vi "open_project_Dialog.vi"(8 "error in (no error)":cluster{"状态":bool, "代码":i32, "源":string} caption="错误输入（无错误）", 11 "当前项目配置 输入":T1) -> (0 "error out":cluster{"状态":bool, "代码":i32, "源":string} caption="错误输出", 1 "结果":bool, 2 "取消？":bool, 3 "当前项目配置 输出":T1)   [LabVIEW 2018, in "menu.lvlib"]
uses:
  menu.lvlib
panel:
  in  "取消按钮":bool
  in  "确定按钮":bool
  in  "项目文件路径":path
  in  "项目名":string
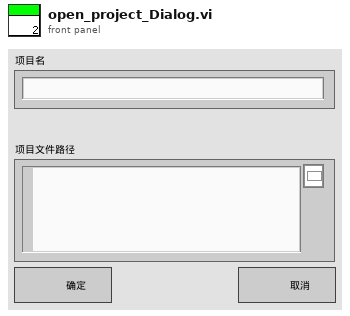
[diagram p1: front panel]
types:
  T1 = cluster{"控制参数配置":string, "模拟响应配置":string, "串口通信配置":string, "数据显示配置":string, "数据记录配置":string, "安全/报警配置":string, "模拟负载数据":string, "模拟加载数据":string, "总电源":bool, "电机1上电":bool, "电机2上电":bool, "串口连接":bool, "电机1\n相电流报警":bool, "电机2\n相电流报警":bool, "电机1\n母线电压报警":bool, "电机2\n母线电压报警":bool, "保存设置":bool, "从文件加载":bool, "恢复默认设置":bool, "路径":path, "项目路径":path, "项目名":string, "创建时间":string, "上次使用时间":string}
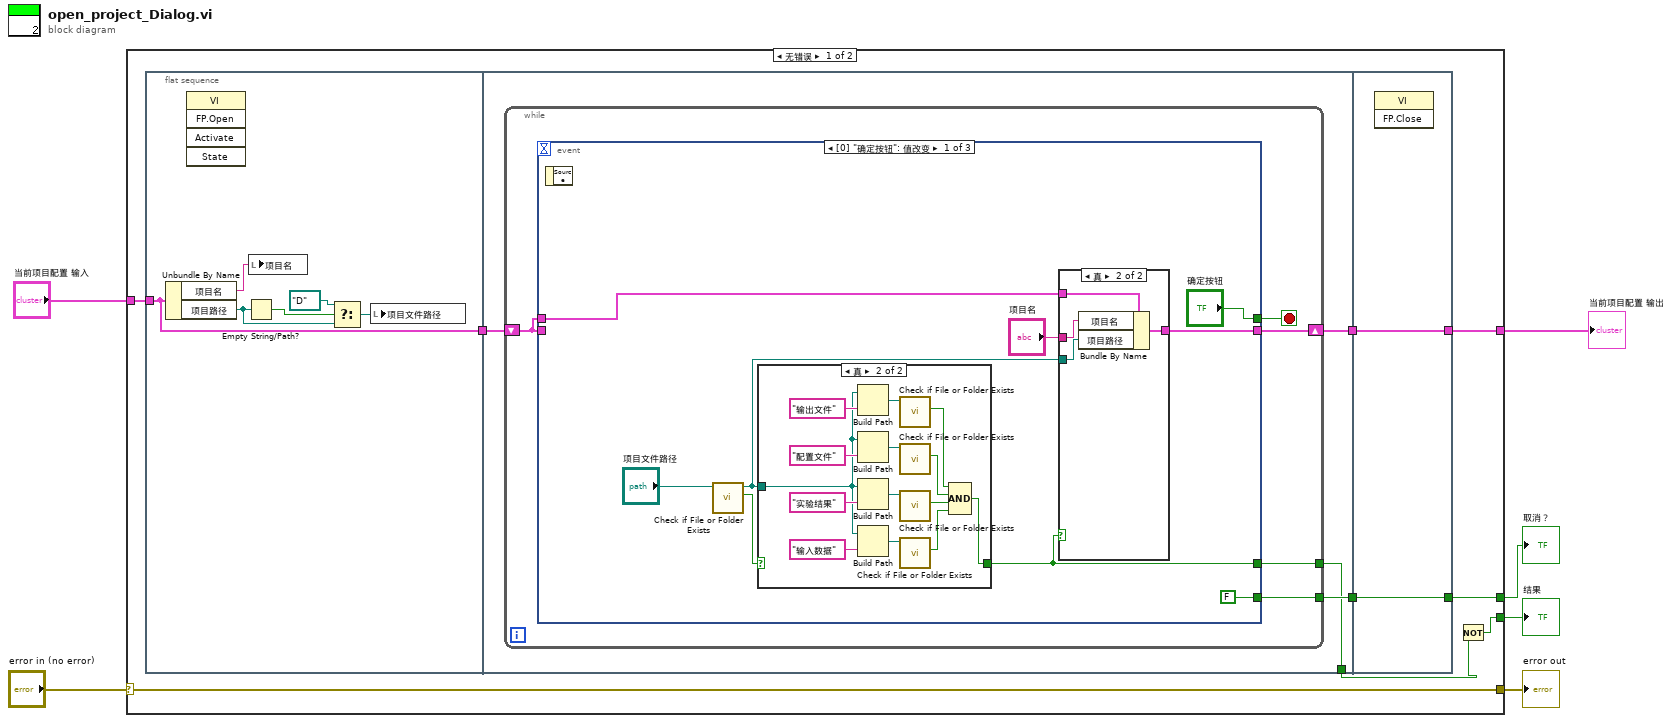
[diagram p0: block diagram]
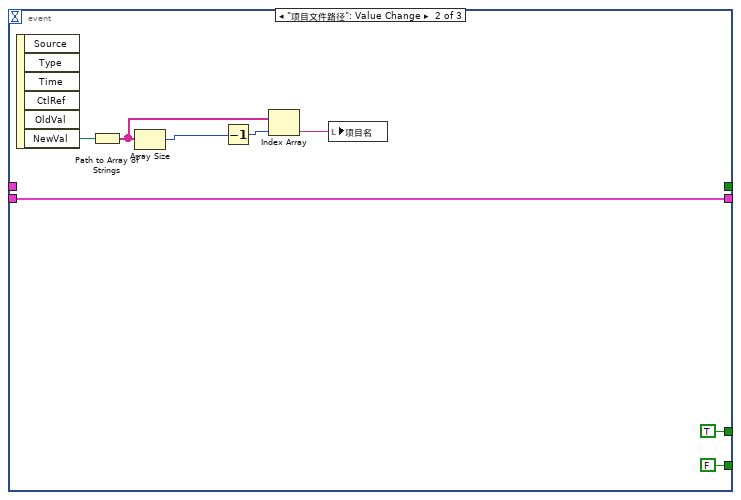
[diagram p4: hidden frame]
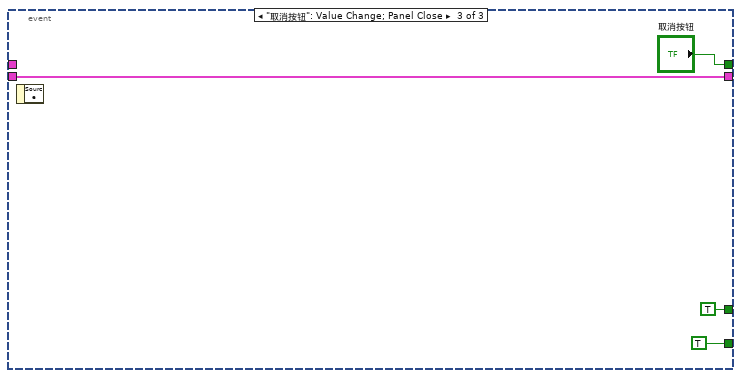
[diagram p5: hidden frame]
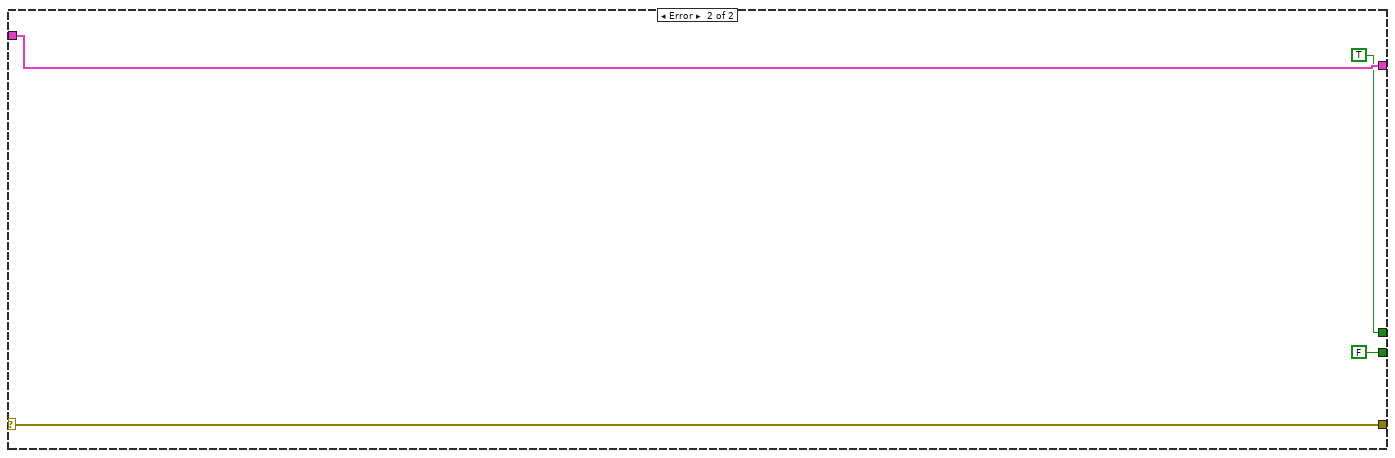
[diagram p6: hidden frame]
diagram:
  n1 = case shown="无错误" "error in (no error)" {
    selector: "error in (no error)" -> [w15 w77]
    tunnel: [w15 w77] -> w5
    tunnel: "当前项目配置 输入" -> [w9 w76]
    tunnel: [w13 w76] -> w2
    tunnel: [w14 TRUE ("UI Refresh Needed?")] -> w4
    tunnel: [w8 FALSE] -> w1
    frame No Error {
      n2 = flat-sequence {
        tunnel: w9 -> [w21]
        tunnel: [w21] -> w12
        tunnel: w12 -> [w22]
        tunnel: [w25] -> w11
        tunnel: [w24] -> w10
        tunnel: [w23] -> w7
        tunnel: [w72] -> w13
        tunnel: [w73] -> w14
        tunnel: w11 -> [w73]
        tunnel: w10 -> [w72]
        frame #0 {
          n3 = Unbundle By Name(w21) -> ("项目名"=w20:string, "项目路径"=w18:path)
          n4 = invoke class="VI" method="FP.Open"() -> ()  [unwired: 5 in, 5 out]
          n5 = Empty String/Path?(string/path=w18) -> (empty?=w19:bool)
          n6 = local write "项目名"(w20) -> ()
          n7 = Select(t=path "D:/", s=w19, f=w18) -> (s? t:f=w16:path)
          n8 = local write "项目文件路径"(w16) -> ()
        }
        frame #1 {
          n9 = while {
            tunnel: [w30] -> w25
            tunnel: [w28] -> w23
            shift-right: [w29] -> w24
            shift-left: w22 -> [w27]
            stop <- w26 stop-if-true
            n10 = event shown="[0] \"确定按钮\": 值改变" {
              selector: _ -> [_ _ _]
              dyn-events: _ -> [_ _ _]
              timeout: _ -> [_ _ _]
              tunnel: [w33 w67 w71] -> w29
              tunnel: w27 -> [_ w67 w71]
              tunnel: [FALSE ("UI Refresh Needed?") FALSE ("UI Refresh Needed?") TRUE ("UI Refresh Needed?")] -> w30
              tunnel: [w37 TRUE TRUE] -> w28
              tunnel: w27 -> [w36 _ _]
              tunnel: ["确定按钮" _ "取消按钮"] -> w26
              event "确定按钮": Value Change {
                n11 = event-data() -> ()  [unwired: 1 in, 1 out]
                n12 = call <vilib>:"Check if File or Folder Exists.vi"("path"="项目文件路径") -> ("file or folder exists?"=w38:bool, "dup path"=w34:path)  [unwired: 8 in, 1 out]
                n13 = case shown="真" w38 {
                  selector: w38 -> [w45 _]
                  tunnel: [w45 w47] -> w37
                  tunnel: w34 -> [_ w46]
                  frame False {
                  }
                  frame True {
                    n14 = Build Path(base path=w46, name or relative path="输出文件") -> (appended path=w58:path)
                    n15 = Build Path(base path=w46, name or relative path="配置文件") -> (appended path=w59:path)
                    n16 = Build Path(base path=w46, name or relative path="实验结果") -> (appended path=w57:path)
                    n17 = Build Path(base path=w46, name or relative path="输入数据") -> (appended path=w55:path)
                    n18 = call <vilib>:"Check if File or Folder Exists.vi"("path"=w58) -> ("file or folder exists?"=w51:bool)  [unwired: 8 in, 2 out]
                    n19 = call <vilib>:"Check if File or Folder Exists.vi"("path"=w59) -> ("file or folder exists?"=w50:bool)  [unwired: 8 in, 2 out]
                    n20 = call <vilib>:"Check if File or Folder Exists.vi"("path"=w57) -> ("file or folder exists?"=w49:bool)  [unwired: 8 in, 2 out]
                    n21 = call <vilib>:"Check if File or Folder Exists.vi"("path"=w55) -> ("file or folder exists?"=w48:bool)  [unwired: 8 in, 2 out]
                    n22 = Compound Arithmetic op=AND ("复合运算")(w51, w50, w49, w48) -> (w47:bool)
                  }
                }
                n23 = case shown="真" w37 {
                  tunnel: w36 -> [w40 w44]
                  tunnel: "项目名" -> [_ w43]
                  tunnel: w34 -> [_ w42]
                  tunnel: [w40 w41] -> w33
                  frame False {
                  }
                  frame True {
                    n24 = Bundle By Name(cluster=w44, "项目名"=w43, "项目路径"=w42) -> (w41:T1)
                  }
                }
              }
              event "项目文件路径": Value Change {
                n25 = event-data() -> ("NewVal"=w66:path)  [unwired: 1 in, 5 out]
                n26 = Path to Array of Strings(0:w66) -> (2:w63:string[])  [unwired: 1 out]
                n27 = Array Size(array=w63) -> (size(s)=w65:i32)
                n28 = Decrement(x=w65) -> (x-1=w62:i32)
                n29 = Index Array(array=w63, index=w62) -> (element=w64:string)
                n30 = local write "项目名"(w64) -> ()
              }
              event "取消按钮": Value Change; Panel Close {
                n31 = event-data() -> ()  [unwired: 1 in, 1 out]
              }
            }
          }
        }
        frame #2 {
          n32 = invoke class="VI" method="FP.Close"() -> ()  [unwired: 3 in, 3 out]
        }
      }
      n33 = Not(x=w7) -> (.not. x?=w8:bool)
    }
    frame Error {
    }
  }
  "error out" <- w5
  "取消？" <- w4
  "当前项目配置 输出" <- w2
  "结果" <- w1
